vi "Ref_Num_Combine_Full_Report.vi"(3 "Temporary test data":refnum<vi>, 6 "XY Graph NEW":refnum<vi>, 8 "error in (no error)":errorcluster, 11 "Report Array Header":refnum<vi>) -> (0 "error out":errorcluster)   [LabVIEW 2020]
uses:
  <vilib>/Utility/NIReport.llb/Report Type.ctl
  <vilib>/Utility/file.llb/Read Delimited Spreadsheet (DBL).vi
  <vilib>/Utility/NIReport.llb/NI_report.lvclass
  <vilib>/Utility/NIReport.llb/NI_ReportGenerationCore.lvlib
  <vilib>/Utility/NIReport.llb/Excel/NI_Excel.lvclass
panel:
  out "Report_Header":string[](array[string])
  out "Dual Bias (Index : 14)":string
  out "Compensation (Index : 13)":string
  out "Test Fixture (Index : 6)":string
  out "SheetName":string
  out "Target Test Signal Level":string
  out "Test Type SHORTCUT":string
  out "Measured Test Signal Level":string
  out "REQUEST NUMBER ONLY":string
  out "Test Comment (Index : 12)":string
  out "Lot/Date Code (Index : 11)":string
  out "Lot Number (Index : 10)":string
  out "Capacitance Units (Index : 9)":string
  out "Full Test Signal Level (Index : 8)":string
  out "Test Frequency (Index : 7)":string
  out "Test System (Index : 5)":string
  out "Test Type (Index : 4)":string
  out "Part Number (Index : 3)":string
  out "Date (Index : 2)":string
  out "Request Number (Index : 1)":string
  out "Operator (Index : 0)":string
  # "In Refnum_VRMS"
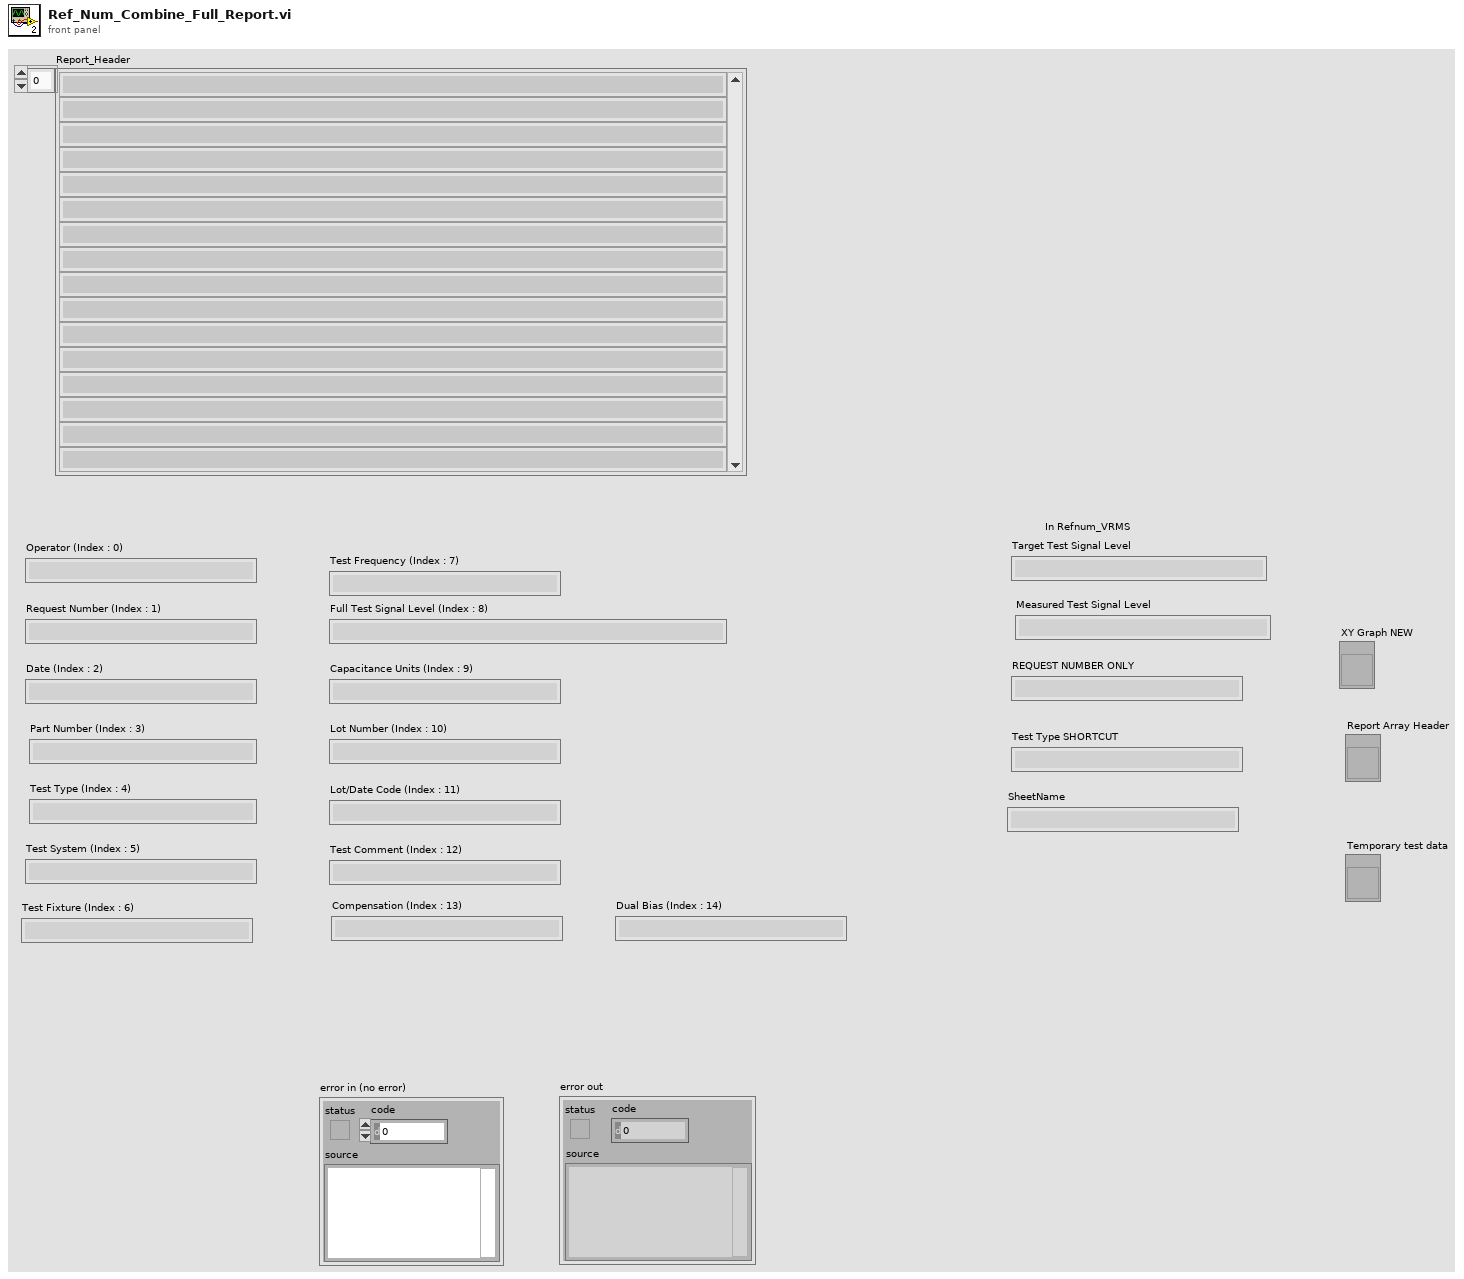
[diagram p1: front panel]
types:
  T1 = enum16{"maximized", "minimized", "normal", "no change"}
  T2 = typedef "NI_ReportGenerationCore.lvlib/Report Type.ctl" = enum16{"HTML", "Word", "Excel"}
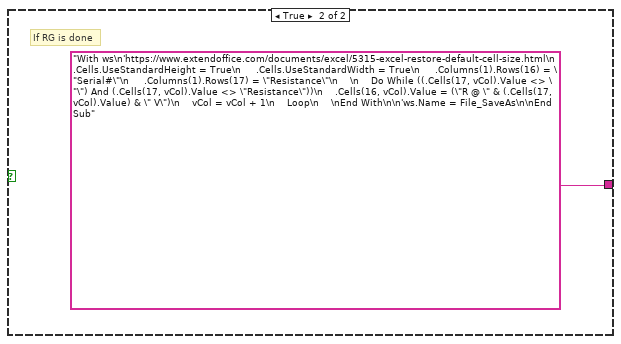
[diagram p3: hidden frame]
diagram:
  n1 = disable-structure shown="Enabled" {
    frame Enabled {
      w24 = ""
      n2 = local write "Full Test Signal Level (Index : 8)"(w24) -> ()
      n3 = local write "REQUEST NUMBER ONLY"(w24) -> ()
      n4 = local write "Lot Number (Index : 10)"(w24) -> ()
      n5 = local write "Measured Test Signal Level"(w24) -> ()
      n6 = local write "Lot/Date Code (Index : 11)"(w24) -> ()
      n7 = local write "Test Comment (Index : 12)"(w24) -> ()
      n8 = local write "Compensation (Index : 13)"(w24) -> ()
      n9 = local write "Dual Bias (Index : 14)"(w24) -> ()
      n10 = local write "Capacitance Units (Index : 9)"(w24) -> ()
      n11 = local write "Test System (Index : 5)"(w24) -> ()
      n12 = local write "Test Frequency (Index : 7)"(w24) -> ()
      n13 = local write "Test Fixture (Index : 6)"(w24) -> ()
      n14 = local write "Part Number (Index : 3)"(w24) -> ()
      n15 = local write "Test Type (Index : 4)"(w24) -> ()
      n16 = local write "Target Test Signal Level"(w24) -> ()
      n17 = local write "Operator (Index : 0)"(w24) -> ()
      n18 = local write "Request Number (Index : 1)"(w24) -> ()
      n19 = local write "Date (Index : 2)"(w24) -> ()
      n20 = local write "Test Type SHORTCUT"(w24) -> ()
      n21 = local write "Report_Header"(string[] ["", "", "", "", "", "", "", "", "", "", "", "", "", "", ""] ("Report Array Header")) -> ()
      n22 = local write "SheetName"(w24) -> ()
    }
    frame Disabled {
    }
  }
  n23 = flat-sequence {
    tunnel: ["error in (no error)"] -> w3
    tunnel: [w35] -> w5
    tunnel: w3 -> [w35]
    tunnel: [w85] -> w4
    tunnel: w5 -> [w86]
    tunnel: w4 -> [w91]
    tunnel: [w90] -> w23
    tunnel: [w89] -> w22
    tunnel: w23 -> [w106]
    tunnel: [w102] -> w21
    tunnel: w22 -> [w105]
    tunnel: [w101] -> w20
    tunnel: [w100] -> w19
    tunnel: w21 -> [w112]
    tunnel: [w110] -> w18
    tunnel: w20 -> [w111]
    tunnel: [w109] -> w17
    tunnel: w19 -> [w108]
    tunnel: w18 -> [w168]
    tunnel: w17 -> [w167]
    tunnel: [w166] -> w16
    tunnel: [w165] -> w15
    tunnel: [w164] -> w14
    tunnel: w16 -> [w178]
    tunnel: w15 -> [w177]
    tunnel: [w176] -> w13
    tunnel: [w175] -> w12
    tunnel: w14 -> [w174]
    tunnel: w13 -> [w190]
    tunnel: [w189] -> w11
    tunnel: w12 -> [w191]
    tunnel: [w192] -> w10
    tunnel: [w188] -> w9
    tunnel: w11 -> [w198]
    tunnel: [w197] -> w8
    tunnel: w10 -> [w200]
    tunnel: [w199] -> w7
    tunnel: w9 -> [w196]
    tunnel: w8 -> [w203]
    tunnel: w7 -> [w202]
    tunnel: [w205] -> w6
    tunnel: w6 -> [w211]
    tunnel: [w210] -> w2
    tunnel: w2 -> [w213]
    tunnel: [w213] -> w1
    tunnel: w1 -> [w217]
    frame #0 {
      w28 = ""
      n24 = local write "Full Test Signal Level (Index : 8)"(w28) -> ()
      n25 = local write "REQUEST NUMBER ONLY"(w28) -> ()
      n26 = local write "Lot Number (Index : 10)"(w28) -> ()
      n27 = local write "Measured Test Signal Level"(w28) -> ()
      n28 = local write "Lot/Date Code (Index : 11)"(w28) -> ()
      n29 = local write "Test Comment (Index : 12)"(w28) -> ()
      n30 = local write "Compensation (Index : 13)"(w28) -> ()
      n31 = local write "Dual Bias (Index : 14)"(w28) -> ()
      n32 = local write "Capacitance Units (Index : 9)"(w28) -> ()
      n33 = local write "Test System (Index : 5)"(w28) -> ()
      n34 = local write "Test Frequency (Index : 7)"(w28) -> ()
      n35 = local write "Test Fixture (Index : 6)"(w28) -> ()
      n36 = local write "Part Number (Index : 3)"(w28) -> ()
      n37 = local write "Test Type (Index : 4)"(w28) -> ()
      n38 = local write "Target Test Signal Level"(w28) -> ()
      n39 = local write "Operator (Index : 0)"(w28) -> ()
      n40 = local write "Request Number (Index : 1)"(w28) -> ()
      n41 = local write "Date (Index : 2)"(w28) -> ()
      n42 = local write "Test Type SHORTCUT"(w28) -> ()
      n43 = local write "Report_Header"(string[] ["", "", "", "", "", "", "", "", "", "", "", "", "", "", ""] ("Report Array Header")) -> ()
      n44 = Wait (ms)(milliseconds to wait=u32 1000 ("millisecond timer value")) -> ()  [unwired: 1 out]
      n45 = local write "SheetName"(w28) -> ()
    }
    frame #1 {
      # "Generate Bitmap from XY Graph,\nAppend graph into XLS file"
      # "TRYOUTS DATA ACQUISITION"
      n46 = property class="Arr (strict)"(reference="Report Array Header") -> ("Value"=w33:string[])  [unwired: 1 in, 2 out]
      n47 = local write "Report_Header"(w33) -> ()
      n48 = Index Array(array=w33, index=12) -> (element=w76:string)
      n49 = Index Array(array=w33, index=13) -> (element=w81:string)
      n50 = Index Array(array=w33, index=9) -> (element=w73:string)
      n51 = Index Array(array=w33, index=10) -> (element=w74:string)
      n52 = Index Array(array=w33, index=11) -> (element=w75:string)
      n53 = Index Array(array=w33, index=7) -> (element=w72:string)
      n54 = Index Array(array=w33, index=8) -> (element=w77:string)
      n55 = Index Array(array=w33, index=14) -> (element=w82:string)
      n56 = Index Array(array=w33, index=5) -> (element=w71:string)
      n57 = Index Array(array=w33, index=6) -> (element=w79:string)
      n58 = Index Array(array=w33, index=1) -> (element=w83:string)
      n59 = Index Array(array=w33, index=2) -> (element=w68:string)
      n60 = Index Array(array=w33, index=3) -> (element=w69:string)
      n61 = Index Array(array=w33, index=4) -> (element=w70:string)
      n62 = Index Array(array=w33, index=0) -> (element=w67:string)
      n63 = local write "Lot Number (Index : 10)"(w74) -> ()
      n64 = local write "Capacitance Units (Index : 9)"(w73) -> ()
      n65 = local write "Lot/Date Code (Index : 11)"(w75) -> ()
      n66 = local write "Test Comment (Index : 12)"(w76) -> ()
      n67 = local write "Compensation (Index : 13)"(w81) -> ()
      n68 = local write "Dual Bias (Index : 14)"(w82) -> ()
      n69 = local write "Test Frequency (Index : 7)"(w72) -> ()
      n70 = local write "Test System (Index : 5)"(w71) -> ()
      n71 = local write "Test Fixture (Index : 6)"(w79) -> ()
      n72 = local write "Part Number (Index : 3)"(w69) -> ()
      n73 = local write "Test Type (Index : 4)"(w70) -> ()
      n74 = local write "Operator (Index : 0)"(w67) -> ()
      n75 = local write "Request Number (Index : 1)"(w83) -> ()
      n76 = local write "Date (Index : 2)"(w68) -> ()
      n77 = call-poly <vilib>:"Read Delimited Spreadsheet.vi"("file path (dialog if empty)"=path "C:/Capacitance_Project/Cap_Temp_data/temp_test_data.csv", "delimiter (\\t)"="," ("delimiter (\\t)")) -> ("all rows"=w44:dbl[][])  [unwired: 8 in, 5 out]
      n78 = property class="Arr (strict)"(reference="Temporary test data", "Value"=w44) -> ()  [unwired: 1 in, 2 out]
      n79 = local write "Full Test Signal Level (Index : 8)"(w77) -> ()
      n80 = Match Pattern(string=w70, regular expression="Test Type: ") -> (after substring=w31:string)  [unwired: 1 in, 3 out]
      n81 = Match Pattern(string=w83, regular expression="Request Number: ") -> (after substring=w84:string)  [unwired: 1 in, 3 out]
      n82 = invoke class="XYGraph (strict)" method="Export Image"(reference="XY Graph NEW", "FileType"=enum32{"BMP", "EPS", "EMF", "PICT"}."BMP" ("File Type"), "Target"=enum32{"File", "Clipboard"}."File", "Path"=path "C:/Capacitance_Project/Cap_Temp_data/temp_chart.bmp", "HideGrid"=FALSE ("Hide Grid"), "Overwrite"=TRUE ("Always Overwrite")) -> ()  [unwired: 2 in, 8 out]
      n83 = String Subset(string=w31, length (rest)=3 ("length (rest)")) -> (substring=w30:string)  [unwired: 1 in]
      n84 = local write "REQUEST NUMBER ONLY"(w84) -> ()
      n85 = local write "Test Type SHORTCUT"(w30) -> ()
      n86 = Concatenate Strings(w84, w30) -> (w78:string)
      n87 = Match Pattern(string=w77, regular expression=",") -> (after substring=w66:string)  [unwired: 1 in, 3 out]
      n88 = Match Pattern(string=w77, regular expression=",") -> (before substring=w65:string)  [unwired: 1 in, 3 out]
      n89 = local write "SheetName"(w78) -> ()
      n90 = Wait (ms)(milliseconds to wait=u32 3000 ("millisecond timer value")) -> ()  [unwired: 1 out]
      n91 = local write "Measured Test Signal Level"(w66) -> ()
      n92 = local write "Target Test Signal Level"(w65) -> ()
    }
    frame #2 {
      n93 = call "Message_dialog.vi"("error in (no error)"=w86, "set delay"=3.0, "String"="GENERATING REPORT\n......................................\n\n\nPLEASE WAIT for 15 seconds " ("Message")) -> ("error out"=w85:errorcluster)  [unwired: 8 in]
    }
    frame #3 {
      n94 = call <vilib>:"Create Report.vi"("window state (normal)"=T1."maximized", "report type"=Report_Type."Excel", "error in (no error)"=w91) -> ("report out"=w94:refnum<class "NI_report.lvclass">, "error out"=w95:errorcluster)  [unwired: 11 in]
      n95 = Wait (ms)(milliseconds to wait=u32 300 ("millisecond timer value")) -> ()  [unwired: 1 out]
      n96 = call <vilib>:"Excel Bring to Front.vi"("report in"=w94, "window state (maximized)"=enum16{"maximized", "minimized", "normal"}."maximized", "error in (no error)"=w95) -> ("report out"=w90:refnum<class "NI_report.lvclass">, "error out"=w89:errorcluster)  [unwired: 11 in]
    }
    frame #4 {
      n97 = call <vilib>:"Excel Import Module.vi"("report in"=w106, "module code (\"\")"="Sub InsertImage()\n\n\nDim ws As Worksheet\nDim imagePath As String\nDim imgLeft As Double\nDim imgTop As Double\nDim s As String\n\nSet ws = ActiveSheet\ns = \"J1\"\nimagePath = \"C:\\Capacitance_Project\\Cap_Temp_data\\temp_chart.bmp\"\nimgLeft = Range(s).Left\nimgTop = Range(s).Top\n\n'Width & Height = -1 means keep original size\nws.Shapes.AddPicture _\n    fileName:=imagePath, _\n    LinkToFile:=msoFalse, _\n    SaveWithDocument:=msoTrue, _\n    Left:=imgLeft, _\n    Top:=imgTop, _\n    Width:=380, _\n    Height:=218\n\nEnd Sub\n" ("module code (\"\")"), "error in (no error)"=w105) -> ("report out"=w103:refnum<class "NI_report.lvclass">, "module reference"=w100:refnum<k7>, "error out"=w104:errorcluster)  [unwired: 10 in]
      n98 = call <vilib>:"Excel Run Macro.vi"("report in"=w103, "macro name"="InsertImage", "error in (no error)"=w104) -> ("report out"=w102:refnum<class "NI_report.lvclass">, "error out"=w101:errorcluster)  [unwired: 10 in, 1 out]
      n99 = Wait (ms)(milliseconds to wait=u32 300 ("millisecond timer value")) -> ()  [unwired: 1 out]
    }
    frame #5 {
      n100 = call <vilib>:"Excel Remove Module.vi"("report in"=w112, "module reference"=w108, "error in (no error)"=w111) -> ("report out"=w110:refnum<class "NI_report.lvclass">, "error out"=w109:errorcluster)  [unwired: 11 in]
      n101 = Wait (ms)(milliseconds to wait=u32 300 ("millisecond timer value")) -> ()  [unwired: 1 out]
    }
    frame #6 {
      w157 = "\""
      w158 = "\r\n"
      n102 = local read "Test Type (Index : 4)"() -> (w160:string)
      n103 = Match Pattern(string=w160, regular expression="Test Type: ") -> (after substring=w161:string)  [unwired: 1 in, 3 out]
      n104 = Equal?(x=w161, y="RG") -> (x = y?=w115:bool)
      n105 = case shown="False" w115 {
        tunnel: ["With ws\n'https://www.extendoffice.com/documents/excel/5315-excel-restore-default-cell-size.html\n     .Cells.UseStandardHeight = True\n     .Cells.UseStandardWidth = True\n     .Columns(1).Rows(16) = \"Serial#\"\n     .Columns(1).Rows(17) = \"Capacitance\"\n    \n    Do While ((.Cells(17, vCol).Value <> \"\") And (.Cells(17, vCol).Value <> \"Capacitance\"))\n    .Cells(16, vCol).Value = (\"C @ \" & (.Cells(17, vCol).Value) & \" V\")\n    vCol = vCol + 1\n    Loop\n    \nEnd With\n\n'ws.Name = File_SaveAs\n\nEnd Sub" ("string") "With ws\n'https://www.extendoffice.com/documents/excel/5315-excel-restore-default-cell-size.html\n     .Cells.UseStandardHeight = True\n     .Cells.UseStandardWidth = True\n     .Columns(1).Rows(16) = \"Serial#\"\n     .Columns(1).Rows(17) = \"Resistance\"\n    \n    Do While ((.Cells(17, vCol).Value <> \"\") And (.Cells(17, vCol).Value <> \"Resistance\"))\n    .Cells(16, vCol).Value = (\"R @ \" & (.Cells(17, vCol).Value) & \" V\")\n    vCol = vCol + 1\n    Loop\n    \nEnd With\n\n'ws.Name = File_SaveAs\n\nEnd Sub" ("string")] -> w114
        frame False {
        }
        frame True {
          # "If RG is done"
        }
      }
      n106 = local read "Full Test Signal Level (Index : 8)"() -> (w137:string)
      n107 = local read "Request Number (Index : 1)"() -> (w120:string)
      n108 = local read "Capacitance Units (Index : 9)"() -> (w139:string)
      n109 = local read "Compensation (Index : 13)"() -> (w151:string)
      n110 = local read "Lot/Date Code (Index : 11)"() -> (w143:string)
      n111 = local read "Test Frequency (Index : 7)"() -> (w135:string)
      n112 = local read "Test Comment (Index : 12)"() -> (w145:string)
      n113 = local read "REQUEST NUMBER ONLY"() -> (w147:string)
      n114 = local read "Test Type SHORTCUT"() -> (w149:string)
      n115 = local read "Part Number (Index : 3)"() -> (w124:string)
      n116 = local read "Lot Number (Index : 10)"() -> (w141:string)
      n117 = local read "Test System (Index : 5)"() -> (w131:string)
      n118 = local read "Test Fixture (Index : 6)"() -> (w133:string)
      n119 = local read "Dual Bias (Index : 14)"() -> (w153:string)
      n120 = local read "Test Type (Index : 4)"() -> (w126:string)
      n121 = local read "Operator (Index : 0)"() -> (w118:string)
      n122 = local read "Date (Index : 2)"() -> (w122:string)
      n123 = local read "SheetName"() -> (w156:string)
      n124 = Concatenate Strings(w158, "Operator = \"", w118, w157, w158, "Request_Number = \"" ("string"), w120, w157, w158, "Curr_Date = \"" ("string"), w122, w157, w158, "Part_Number = \"" ("string"), w124, w157, w158, "Test_Type = \"" ("string"), w126, w157, w158, "Test_System = \"" ("string"), w131, w157, w158, "Test_Fixture = \"", w133, w157, w158, "Test_Frequency = \"" ("string"), w135, w157, w158, "Test_Signal_Level = \"" ("string"), w137, w157, w158, "Capacitance_Units = \"" ("string"), w139, w157, w158, "Lot_Number = \"" ("string"), w141, w157, w158, "Lot_Date = \"" ("string"), w143, w157, w158, "Test_Comment = \"" ("string"), w145, w157, w158, "REQUEST_NUM_ONLY = \"" ("string"), w147, w157, w158, "TEST_TYPE_SHORTFORM = \"" ("string"), w149, w157, w158, "Compensation = \"" ("string"), w151, w157, w158, "DualBias = \"" ("string"), w153, w157, w158, "File_SaveAs = \"" ("string"), w156, w157, w158) -> (w128:string)
      n125 = Concatenate Strings("Sub Step1()\n\nDim Operator As String\nDim Request_Number As String\nDim Curr_Date As String\nDim Part_Number As String\nDim Test_Type As String\nDim Test_System As String\nDim Test_Fixture As String\nDim Test_Frequency As String\nDim Test_Signal_Level As String\nDim Capacitance_Units As String\nDim Lot_Number As String\nDim Lot_Date As String\nDim Test_Comment As String\nDim Compensation As String\nDim DualBias As String\n\nDim REQUEST_NUM_ONLY As String\nDim TEST_TYPE_SHORTFORM As String\nDim File_SaveAs As String\nDim ws As Worksheet\nDim strFile As String\nDim vCol As Integer\n'-----------------------------------------------------------------\n'must have a space after :_", w128, "vCol = 2\nstrFile = \"C:\\Capacitance_Project\\Cap_Temp_data\\temp_test_data.csv\"\n'-----------------------------------------------------------------\n\nSet ws = ActiveSheet\nws.Select\nws.Activate\nws.Name = File_SaveAs\n\n'-----------------------------------------------------------------\n\nws.Columns(1).Rows(1) = Operator\nws.Columns(1).Rows(2) = Request_Number\nws.Columns(1).Rows(3) = Curr_Date\nws.Columns(1).Rows(4) = Part_Number\nws.Columns(1).Rows(5) = Test_Type\nws.Columns(1).Rows(6) = Test_System\nws.Columns(1).Rows(7) = Test_Fixture \nws.Columns(1).Rows(8) = Test_Frequency\nws.Columns(1).Rows(9) = Test_Signal_Level\nws.Columns(1).Rows(10) = Capacitance_Units\nws.Columns(1).Rows(11) = Lot_Number\nws.Columns(1).Rows(12) = Lot_Date\nws.Columns(1).Rows(13) = Test_Comment\nws.Columns(1).Rows(14) = Compensation\nws.Columns(1).Rows(15) = DualBias\n\n'-----------------------------------------------------------------\n\n'-----------------------------------------------------------------\n''https://stackoverflow.com/questions/12197274/is-there-a-way-to-import-data-from-csv-to-active-excel-sheet\nWith ws.QueryTables.Add(Connection:=\"TEXT;\" & strFile, Destination:=ws.Range(\"A17\"))\n     .TextFileParseType = xlDelimited\n     .TextFileCommaDelimiter = True\n     .Refresh\nEnd With\n" ("module code (\"\")"), w114) -> (w116:string)
      n126 = call <vilib>:"Excel Import Module.vi"("report in"=w168, "module code (\"\")"=w116, "error in (no error)"=w167) -> ("report out"=w170:refnum<class "NI_report.lvclass">, "module reference"=w164:refnum<k7>, "error out"=w169:errorcluster)  [unwired: 10 in]
      n127 = call <vilib>:"Excel Run Macro.vi"("report in"=w170, "macro name"="Step1", "error in (no error)"=w169) -> ("report out"=w166:refnum<class "NI_report.lvclass">, "error out"=w165:errorcluster)  [unwired: 10 in, 1 out]
      n128 = Wait (ms)(milliseconds to wait=u32 300 ("millisecond timer value")) -> ()  [unwired: 1 out]
    }
    frame #7 {
      n129 = call <vilib>:"Excel Remove Module.vi"("report in"=w178, "module reference"=w174, "error in (no error)"=w177) -> ("report out"=w176:refnum<class "NI_report.lvclass">, "error out"=w175:errorcluster)  [unwired: 11 in]
      n130 = Wait (ms)(milliseconds to wait=u32 300 ("millisecond timer value")) -> ()  [unwired: 1 out]
    }
    frame #8 {
      w184 = "\r\n"
      n131 = local read "SheetName"() -> (w186:string)
      n132 = Wait (ms)(milliseconds to wait=u32 300 ("millisecond timer value")) -> ()  [unwired: 1 out]
      n133 = Concatenate Strings(w184, "SheetName1 = \"" ("string"), w186, "\"", w184) -> (w185:string)
      n134 = Concatenate Strings("Sub Step2()\n\n\nDim SheetName1 As String\n", w185, "\n'-----------------------------------------------------------------\n\n'Variable declaration\n    Dim wb As Workbook\n   \n    'Create New Workbook\n    Set wb = Workbooks.Add\n\n    'Save Above Created New Workbook\n    Dim relativePath As String\n    relativePath = \"C:\\Capacitance_Project\" & \"\\\" & SheetName1 & \".xls\"\n    \n    wb.SaveAs Filename:=relativePath\n                  \nThisWorkbook.Sheets(SheetName1).Copy Before:=wb.Sheets(Sheets.Count) \n\n'----------------------------------------------------------\n\tDim FINDws As Worksheet\n\tDim mySheet As Variant\n\t\n\tmySheet = SheetName1\n\nFor Each FINDws In wb.Worksheets\n    If mySheet <> FINDws.Name Then\n      FINDws.Delete\n    End If\nNext FINDws \n\nwb.Save\nwb.Close            \n\n\nEnd Sub" ("module code (\"\")")) -> (w179:string)
      n135 = call <vilib>:"Excel Import Module.vi"("report in"=w190, "module code (\"\")"=w179, "error in (no error)"=w191) -> ("report out"=w193:refnum<class "NI_report.lvclass">, "module reference"=w188:refnum<k7>, "error out"=w194:errorcluster)  [unwired: 10 in]
      n136 = call <vilib>:"Excel Run Macro.vi"("report in"=w193, "macro name"="Step2", "error in (no error)"=w194) -> ("report out"=w189:refnum<class "NI_report.lvclass">, "error out"=w192:errorcluster)  [unwired: 10 in, 1 out]
    }
    frame #9 {
      n137 = call <vilib>:"Excel Remove Module.vi"("report in"=w198, "module reference"=w196, "error in (no error)"=w200) -> ("report out"=w197:refnum<class "NI_report.lvclass">, "error out"=w199:errorcluster)  [unwired: 11 in]
      n138 = Wait (ms)(milliseconds to wait=u32 300 ("millisecond timer value")) -> ()  [unwired: 1 out]
    }
    frame #10 {
      n139 = Wait (ms)(milliseconds to wait=u32 300 ("millisecond timer value")) -> ()  [unwired: 1 out]
      n140 = call <vilib>:"Excel Bring to Front.vi"("report in"=w203, "window state (maximized)"=enum16{"maximized", "minimized", "normal"}."maximized", "error in (no error)"=w202) -> ("report out"=w207:refnum<class "NI_report.lvclass">, "error out"=w206:errorcluster)  [unwired: 11 in]
      n141 = call-dynamic "Dispose Report.vi"("report in"=w207, "error in (no error)"=w206) -> ("error out"=w205:errorcluster)  [unwired: 13 in]
    }
    frame #11 {
      n142 = call "Message_dialog.vi"("error in (no error)"=w211, "set delay"=2.0, "String"="- Finish - " ("Message")) -> ("error out"=w210:errorcluster)  [unwired: 8 in]
    }
    frame #12 {
      w214 = ""
      n143 = local write "Full Test Signal Level (Index : 8)"(w214) -> ()
      n144 = local write "REQUEST NUMBER ONLY"(w214) -> ()
      n145 = local write "Lot Number (Index : 10)"(w214) -> ()
      n146 = local write "Measured Test Signal Level"(w214) -> ()
      n147 = local write "Lot/Date Code (Index : 11)"(w214) -> ()
      n148 = local write "Test Comment (Index : 12)"(w214) -> ()
      n149 = local write "Compensation (Index : 13)"(w214) -> ()
      n150 = local write "Dual Bias (Index : 14)"(w214) -> ()
      n151 = local write "Capacitance Units (Index : 9)"(w214) -> ()
      n152 = local write "Test System (Index : 5)"(w214) -> ()
      n153 = local write "Test Frequency (Index : 7)"(w214) -> ()
      n154 = local write "Test Fixture (Index : 6)"(w214) -> ()
      n155 = local write "Part Number (Index : 3)"(w214) -> ()
      n156 = local write "Test Type (Index : 4)"(w214) -> ()
      n157 = local write "Target Test Signal Level"(w214) -> ()
      n158 = local write "Operator (Index : 0)"(w214) -> ()
      n159 = local write "Request Number (Index : 1)"(w214) -> ()
      n160 = local write "Date (Index : 2)"(w214) -> ()
      n161 = local write "Test Type SHORTCUT"(w214) -> ()
      n162 = local write "Report_Header"(string[] ["", "", "", "", "", "", "", "", "", "", "", "", "", "", ""] ("Report Array Header")) -> ()
      n163 = Wait (ms)(milliseconds to wait=u32 1000 ("millisecond timer value")) -> ()  [unwired: 1 out]
      n164 = local write "SheetName"(w214) -> ()
    }
    frame #13 {
      "error out" <- w217
    }
  }
